vi "Set Relative Path.vi"(1 "Application Relative Path":string) -> (0 "Full Path":path)   [LabVIEW 2020, in "gRPC Scripting Tools.lvlib"]
uses:
  gRPC Scripting Tools.lvlib
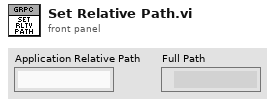
[diagram p1: front panel]
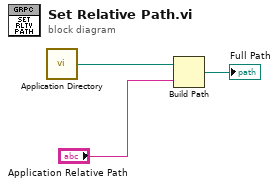
[diagram p0: block diagram]
diagram:
  n1 = call <vilib>:"Application Directory.vi"() -> ("Application Directory"=w1:path)
  n2 = Build Path(base path=w1, name or relative path="Application Relative Path") -> (appended path=→"Full Path":path)
